vi "Display_LookUpScoreRGB.vi"(3 "Position":T2, 4 "ActivePixel":T3, 8 "Player":T1) -> (15 "Draw":bool, 16 "Red":bool, 17 "Green":bool, 18 "Blue":bool)   [LabVIEW 2018]
uses:
  TypDefs/ActivePixel_Cluster.ctl
  FPGA VGA Graphics/FPGA VGA Library/TypDefs/VGA_Position.ctl
  TypDefs/Player_Enum.ctl
  <vilib>/rvi/Memory/Memory_Emulation/nirvimemoryFastEmulation.vi
  <vilib>/rvi/Memory/Memory_Emulation/nirvimemoryEmulation.vi
  <vilib>/rvi/Emulation/niFpgaEmulationIsFPGAContextNoSignature.vi
  <vilib>/rvi/DataTransferAndStorage/Container/Common/niFpgaContainerGetUniqueNameForEmu.vi
  <vilib>/rvi/Emulation/niFpgaProcessEmulError.vi
  <vilib>/rvi/Emulation/niFpgaSctlEmulationGetInTimedLoop.vi
  <vilib>/rvi/errors/nirviReportUnexpectedCaseInternalError (U32).vi
  <vilib>/rvi/DataTransferAndStorage/Container/XNode/niFpgaContainer.xnode
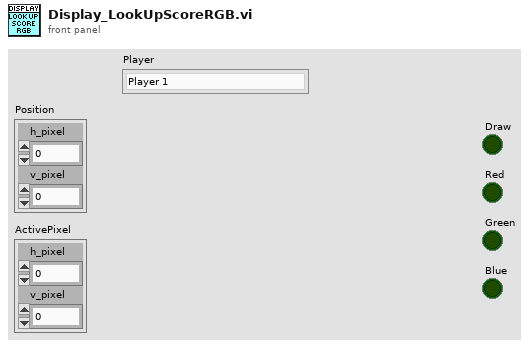
[diagram p1: front panel]
types:
  T1 = typedef "Player_Enum.ctl" = enum16{"Player 1", "Player 2"}
  T2 = typedef "VGA_Position.ctl" = cluster{"h_pixel":i16, "v_pixel":i16}
  T3 = typedef "ActivePixel_Cluster.ctl" = cluster{"h_pixel":i16, "v_pixel":i16}
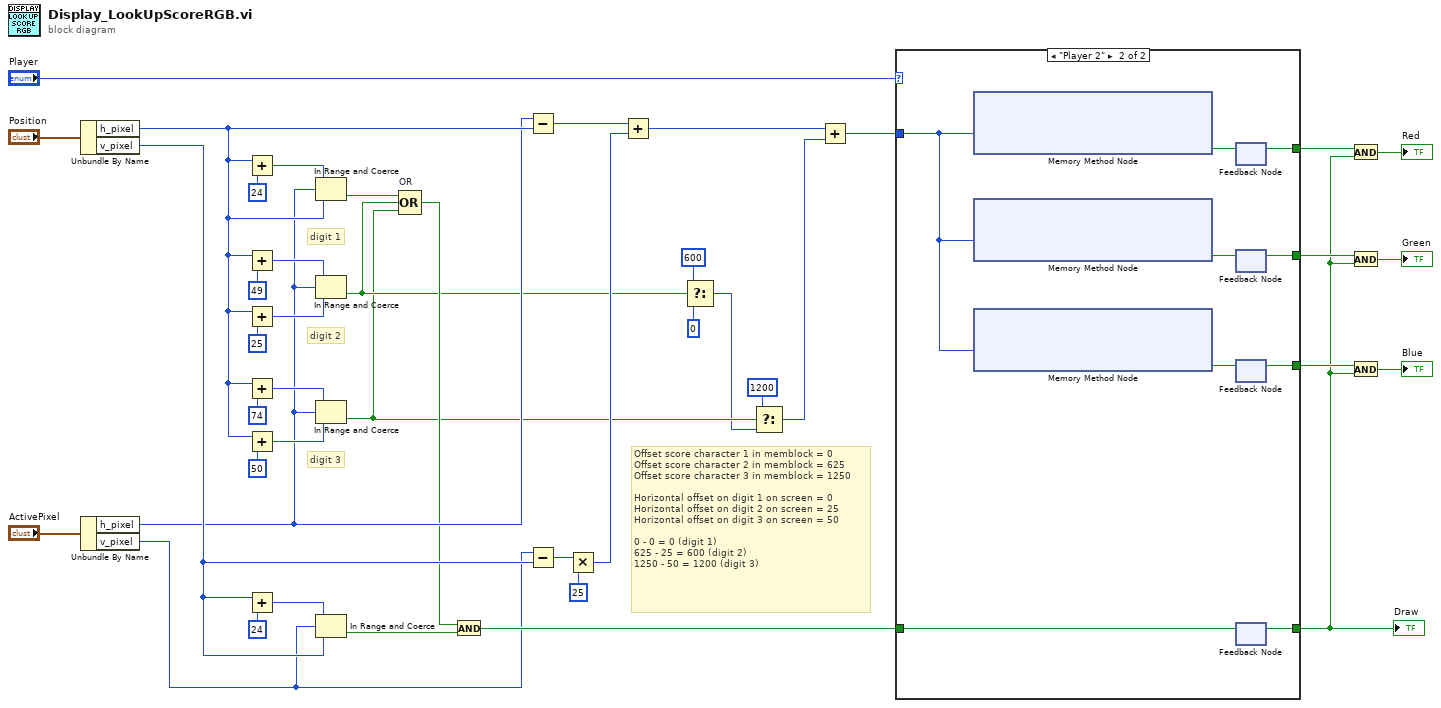
[diagram p0: block diagram]
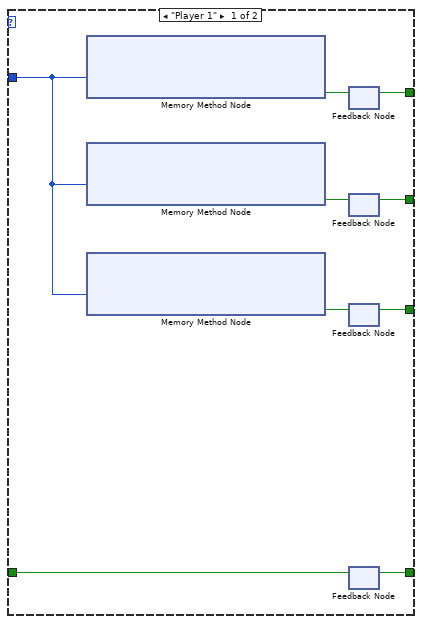
[diagram p2: hidden frame]
diagram:
  # "Offset score character 1 in memblock = 0\nOffset score character 2 in memblock = 625\nOffset score character 3 in memblock = 1250\n\nHorizontal offset on digit 1 on screen = 0\nHorizontal offset on digit 2 on screen = 25\nHorizontal offset on digit 3 on screen = 50\n\n0 - 0 = 0 (digit 1)\n625 - 25 = 600 (digit 2)\n1250 - 50 = 1200 (digit 3)"
  # "digit 3"
  # "digit 2"
  # "digit 1"
  n1 = Unbundle By Name("Position") -> ("h_pixel"=w13:i16, "v_pixel"=w32:i16)
  n2 = Unbundle By Name("ActivePixel") -> ("h_pixel"=w12:i16, "v_pixel"=w31:i16)
  n3 = Add(x=w13, y=i16 24) -> (x+y=w41:i16)
  n4 = Add(x=w13, y=i16 49) -> (x+y=w21:i16)
  n5 = Add(x=w13, y=i16 25) -> (x+y=w18:i16)
  n6 = Add(x=w13, y=i16 74) -> (x+y=w14:i16)
  n7 = Add(x=w13, y=i16 50) -> (x+y=w17:i16)
  n8 = Add(x=w32, y=i16 24) -> (x+y=w40:i16)
  n9 = In Range and Coerce(upper limit=w41, x=w12, lower limit=w13) -> (In Range?=w11:bool)  [unwired: 1 out]
  n10 = In Range and Coerce(upper limit=w21, x=w12, lower limit=w18) -> (In Range?=w9:bool)  [unwired: 1 out]
  n11 = In Range and Coerce(upper limit=w14, x=w12, lower limit=w17) -> (In Range?=w8:bool)  [unwired: 1 out]
  n12 = In Range and Coerce(upper limit=w40, x=w31, lower limit=w32) -> (In Range?=w37:bool)  [unwired: 1 out]
  n13 = Compound Arithmetic op=OR "OR"(w11, w9, w8) -> (w10:bool)
  n14 = And(x=w10, y=w37) -> (x .and. y?=w38:bool)
  n15 = Subtract(x=w12, y=w13) -> (x-y=w39:i16)
  n16 = Subtract(x=w31, y=w32) -> (x-y=w36:i16)
  n17 = Multiply(x=w36, y=i16 25) -> (x*y=w34:i16)
  n18 = Add(x=w39, y=w34) -> (x+y=w23:i16)
  n19 = Select(t=i16 600 ("y"), s=w9, f=i16 0) -> (s? t:f=w7:i16)
  n20 = Select(t=i16 1200 ("y"), s=w8, f=w7) -> (s? t:f=w3:i16)
  n21 = Add(x=w23, y=w3) -> (x+y=w22:i16)
  n22 = case shown="\"Player 2\"" "Player" {
    tunnel: w38 -> [w52 w61]
    tunnel: [w50 w59] -> w29
    tunnel: [w47 w56] -> w28
    tunnel: [w46 w55] -> w27
    tunnel: w22 -> [w45 w54]
    tunnel: [w44 w53] -> w2
    frame "Player 1" {
      n23 = xnode ("Memory Method Node")("Address"=w45) -> ("Data"=w51:bool)  [unwired: 1 in, 1 out]
      n24 = xnode ("Memory Method Node")("Address"=w45) -> ("Data"=w48:bool)  [unwired: 1 in, 1 out]
      n25 = xnode ("Memory Method Node")("Address"=w45) -> ("Data"=w49:bool)  [unwired: 1 in, 1 out]
      n26 = feedback #1() -> (w50:bool)  [unwired: 1 in]
      n27 = feedback-in #1(w51) -> ()
      n28 = feedback #2() -> (w47:bool)  [unwired: 1 in]
      n29 = feedback-in #2(w48) -> ()
      n30 = feedback #3() -> (w46:bool)  [unwired: 1 in]
      n31 = feedback-in #3(w49) -> ()
      n32 = feedback #4() -> (w44:bool)  [unwired: 1 in]
      n33 = feedback-in #4(w52) -> ()
    }
    frame "Player 2" {
      n34 = xnode ("Memory Method Node")("Address"=w54) -> ("Data"=w60:bool)  [unwired: 1 in, 1 out]
      n35 = xnode ("Memory Method Node")("Address"=w54) -> ("Data"=w57:bool)  [unwired: 1 in, 1 out]
      n36 = xnode ("Memory Method Node")("Address"=w54) -> ("Data"=w58:bool)  [unwired: 1 in, 1 out]
      n37 = feedback #5() -> (w59:bool)  [unwired: 1 in]
      n38 = feedback-in #5(w60) -> ()
      n39 = feedback #6() -> (w56:bool)  [unwired: 1 in]
      n40 = feedback-in #6(w57) -> ()
      n41 = feedback #7() -> (w55:bool)  [unwired: 1 in]
      n42 = feedback-in #7(w58) -> ()
      n43 = feedback #8() -> (w53:bool)  [unwired: 1 in]
      n44 = feedback-in #8(w61) -> ()
    }
  }
  "Draw" <- w2
  n45 = And(x=w29, y=w2) -> (x .and. y?=→"Red":bool)
  n46 = And(x=w28, y=w2) -> (x .and. y?=→"Green":bool)
  n47 = And(x=w27, y=w2) -> (x .and. y?=→"Blue":bool)
